vi "FTW-JSON-Keys.vi"(0 "JSON Opject":string, 11 "error in":errorcluster) -> (6 "Keys":string[](array[string]), 8 "Values":string[](array[string]), 15 "error out":errorcluster)   [LabVIEW 2015]
uses:
  FTW-JSON.lvclass
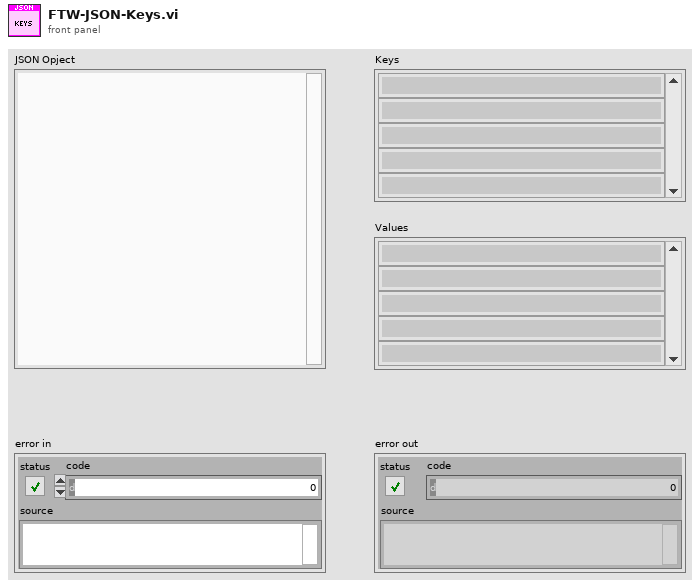
[diagram p1: front panel]
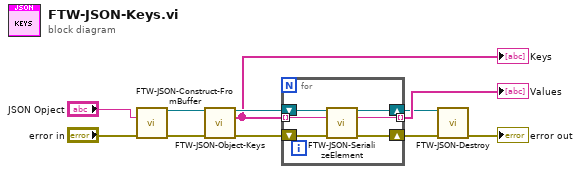
[diagram p0: block diagram]
diagram:
  n1 = call "FTW-JSON-Construct-FromBuffer.vi"("JSON String (UTF-8)"="JSON Opject", "error in"="error in") -> ("JSON Object"=w9:refnum<class "FTW-JSON.lvclass">, "error out"=w8:errorcluster)  [unwired: 12 in]
  n2 = call "FTW-JSON-Object-Keys.vi"("JSON Object"=w9, "error in"=w8) -> ("JSON Object out"=w7:refnum<class "FTW-JSON.lvclass">, "Keys"=w5:string[], "error out"=w6:errorcluster)  [unwired: 11 in]
  "Keys" <- w5
  n3 = for {
    shift-right: [w13] -> w1
    shift-left: w7 -> [w17]
    shift-right: [w12] -> w3
    shift-left: w6 -> [w16]
    tunnel: w5 -> [w15] mode=indexing
    tunnel: [w14] -> w4 mode=indexing
    n4 = call "FTW-JSON-SerializeElement.vi"("JSON Object"=w17, "Key"=w15, "error in"=w16) -> ("JSON Object"=w13:refnum<class "FTW-JSON.lvclass">, "Element as JSON String"=w14:string, "error out"=w12:errorcluster)  [unwired: 9 in, 1 out]
  }
  "Values" <- w4
  n5 = call "FTW-JSON-Destroy.vi"("JSON Object"=w1, "error in"=w3) -> ("error out"=→"error out":errorcluster)  [unwired: 13 in]
